vi "get properties.vi"   [LabVIEW 2020, in "type.lvclass"]
uses:
  type.lvclass
  type.lvclass/type.ctl
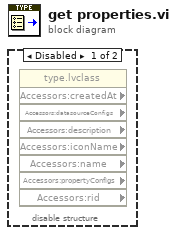
[diagram p0: block diagram]
diagram:
  n1 = disable-structure shown="Disabled" {
    frame Disabled {
      n2 = property class="type.lvclass" props=["Accessors:createdAt", "Accessors:datasourceConfigs", "Accessors:description", "Accessors:iconName", "Accessors:name", "Accessors:propertyConfigs", "Accessors:rid"]() -> ()  [unwired: 2 in, 9 out]
    }
    frame Enabled {
    }
  }
